vi "Compare to Accel Distances.vi"(5 "dA":dbl, 6 "Sample Period (s)":dbl, 7 "Values":cluster{"accel":dbl, "velocity":dbl}, 8 "Speeds in":T1={"maxV (fps)"=20.0, "Accel Limit (fps^2)"=20.0, "Initial V (fps)"=0.0, "Sample Period (s)"=0.02, "Jerk Limit (fps^3)"=0.0, "Distances"=[]}, 9 "Max Robot Speed":dbl, 10 "Current  Length":dbl, 11 "Total Segment Length":dbl) -> (0 "End Loop":bool, 1 "Ends":cluster{"Accel End":bool, "Decel End":bool}, 2 "Values out":cluster{"accel":dbl, "velocity":dbl}, 3 "Action":enum16{"Const", "Accel", "Decel", "Both"}(ring))   [LabVIEW 2025]
uses:
  Types/Speeds.ctl
panel:
  out "Accel Action":enum16{"Const", "Accel", "Decel", "Both"}(ring)
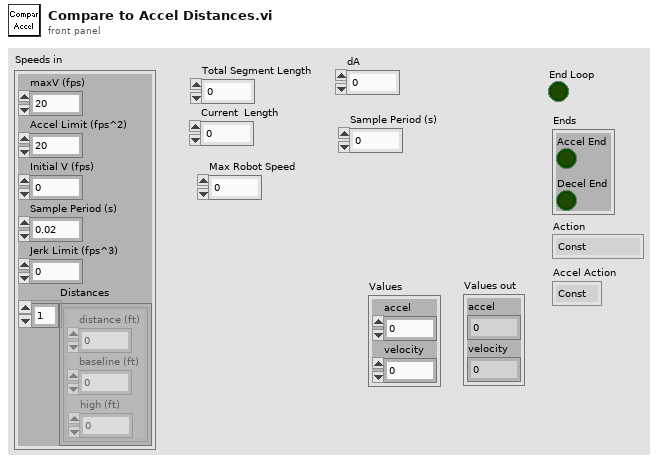
[diagram p1: front panel]
types:
  T1 = typedef "Speeds.ctl" = cluster{"maxV (fps)":dbl, "Accel Limit (fps^2)":dbl, "Initial V (fps)":dbl, "Sample Period (s)":dbl, "Jerk Limit (fps^3)":dbl, "Distances":cluster{"distance (ft)":dbl, "baseline (ft)":dbl, "high (ft)":dbl}[]}
  T2 = cluster{"distance (ft)":dbl, "baseline (ft)":dbl, "high (ft)":dbl}[]
  T3 = cluster{"distance (ft)":dbl, "baseline (ft)":dbl, "high (ft)":dbl}
  T4 = cluster{"distance (ft)":bool, "baseline (ft)":bool, "high (ft)":bool}
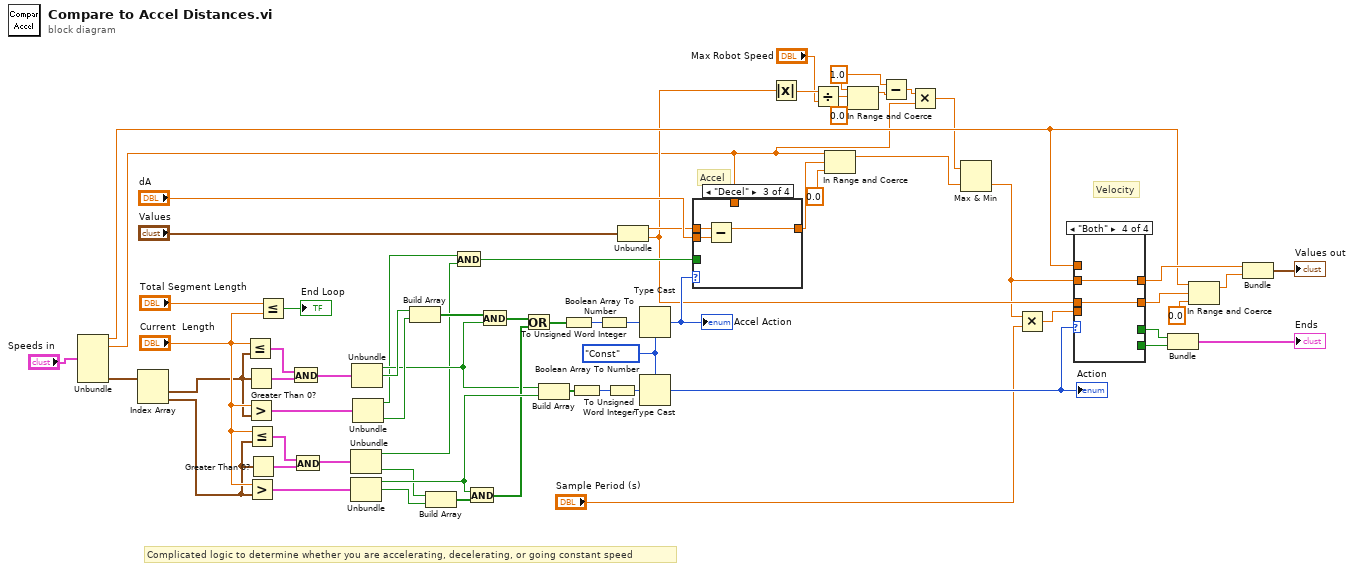
[diagram p0: block diagram]
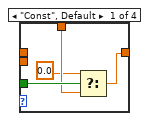
[diagram p2: hidden frame]
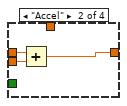
[diagram p3: hidden frame]
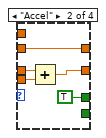
[diagram p6: hidden frame]
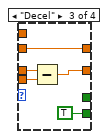
[diagram p7: hidden frame]
diagram:
  w6 = 1.0 ("upper limit")
  w45 = enum16{"Const", "Accel", "Decel", "Both"}."Const" ("Action")
  # "Complicated logic to determine whether you are accelerating, decelerating, or going constant speed"
  # "Accel"
  # "Velocity"
  n1 = Unbundle("Speeds in") -> ("maxV (fps)"=w14:dbl, "Accel Limit (fps^2)"=w4:dbl, "Distances"=w15:T2)  [unwired: 3 out]
  n2 = Index Array(array=w15) -> (element #1=w17:T3, element #2=w16:T3)  [unwired: 2 in]
  n3 = Less Or Equal?(x="Current  Length", y=w17) -> (x <= y?=w62:T4)
  n4 = Greater Than 0?(x=w17) -> (x > 0?=w63:T4)
  n5 = Greater?(x="Current  Length", y=w17) -> (0:w44:T4)
  n6 = Less Or Equal?(x="Current  Length", y=w16) -> (x <= y?=w43:T4)
  n7 = Greater?(x="Current  Length", y=w16) -> (0:w51:T4)
  n8 = Greater Than 0?(x=w16) -> (x > 0?=w42:T4)
  n9 = Less Or Equal?(x="Total Segment Length", y="Current  Length") -> (x <= y?=→"End Loop":bool)
  n10 = And(x=w62, y=w63) -> (x .and. y?=w52:T4)
  n11 = And(x=w43, y=w42) -> (x .and. y?=w39:T4)
  n12 = Unbundle(w39) -> ("distance (ft)"=w19:bool, "high (ft)"=w29:bool)  [unwired: 1 out]
  n13 = Unbundle(w51) -> ("distance (ft)"=w38:bool, "baseline (ft)"=w30:bool)  [unwired: 1 out]
  n14 = Unbundle(w52) -> ("distance (ft)"=w33:bool, "baseline (ft)"=w36:bool)  [unwired: 1 out]
  n15 = Unbundle(w44) -> ("distance (ft)"=w21:bool, "high (ft)"=w40:bool)  [unwired: 1 out]
  n16 = Build Array(w36, w40) -> (w32:bool[])
  n17 = Build Array(w29, w30) -> (w37:bool[])
  n18 = And(x=w21, y=w19) -> (x .and. y?=w20:bool)
  n19 = And(x=w38, y=w37) -> (x .and. y?=w35:bool[])
  n20 = And(x=w32, y=w33) -> (x .and. y?=w31:bool[])
  n21 = Or(x=w31, y=w35) -> (x .or. y?=w34:bool[])
  n22 = Build Array(w33, w38) -> (w53:bool[])
  n23 = Boolean Array To Number(Boolean array=w34) -> (number=w48:u32)
  n24 = Boolean Array To Number(Boolean array=w53) -> (number=w61:u32)
  n25 = To Unsigned Word Integer(number=w48) -> (unsigned 16bit integer=w47:u16)
  n26 = To Unsigned Word Integer(number=w61) -> (unsigned 16bit integer=w50:u16)
  n27 = Unbundle("Values") -> ("accel"=w54:dbl, "velocity"=w12:dbl)
  n28 = Type Cast(type=w45, x=w47) -> (*(type *) &x=w46:enum16{"Const", "Accel", "Decel", "Both"})
  "Accel Action" <- w46
  n29 = Type Cast(type=w45, x=w50) -> (*(type *) &x=w49:enum16{"Const", "Accel", "Decel", "Both"})
  "Action" <- w49
  n30 = case shown="\"Decel\"" w46 {
    tunnel: w54 -> [_ w72 w75 w76]
    tunnel: [w66 w70 w73 w76] -> w24
    tunnel: "dA" -> [_ w71 w74 _]
    tunnel: w4 -> [w68 _ _ _]
    tunnel: w20 -> [w69 _ _ _]
    frame "Const", Default {
      n31 = Select(t=0.0, s=w69, f=w68) -> (s? t:f=w66:dbl)
    }
    frame "Accel" {
      n32 = Add(x=w72, y=w71) -> (x+y=w70:dbl)
    }
    frame "Decel" {
      n33 = Subtract(x=w75, y=w74) -> (x-y=w73:dbl)
    }
    frame "Both" {
    }
  }
  n34 = Absolute Value(x=w12) -> (abs(x)=w11:dbl)
  n35 = Divide(x=w11, y="Max Robot Speed") -> (x/y=w9:dbl)
  n36 = In Range and Coerce(upper limit=w4, x=w24, lower limit=0.0) -> (coerced(x)=w3:dbl)  [unwired: 1 out]
  n37 = In Range and Coerce(upper limit=w6, x=w9, lower limit=0.0) -> (coerced(x)=w7:dbl)  [unwired: 1 out]
  n38 = Subtract(x=w6, y=w7) -> (x-y=w5:dbl)
  n39 = Multiply(x=w5, y=w4) -> (x*y=w2:dbl)
  n40 = Max & Min(x=w2, y=w3) -> (min(x,y)=w1:dbl)  [unwired: 1 out]
  n41 = Multiply(x=w1, y="Sample Period (s)") -> (x*y=w28:dbl)
  n42 = case shown="\"Both\"" w49 {
    tunnel: w12 -> [w77 w83 w88 w90]
    tunnel: [w77 w81 w86 w90] -> w23
    tunnel: w28 -> [_ w82 w87 _]
    tunnel: [_ TRUE _ _] -> w58
    tunnel: [_ _ TRUE _] -> w57
    tunnel: [w78 w79 w84 w89] -> w22
    tunnel: w1 -> [w78 w79 w84 w89]
    tunnel: w14 -> [_ _ _ _]
    frame "Const", Default {
    }
    frame "Accel" {
      n43 = Add(x=w83, y=w82) -> (x+y=w81:dbl)
    }
    frame "Decel" {
      n44 = Subtract(x=w88, y=w87) -> (x-y=w86:dbl)
    }
    frame "Both" {
    }
  }
  n45 = Bundle(w58, w57) -> (→"Ends":cluster{bool, bool})  [unwired: 1 in]
  n46 = In Range and Coerce(upper limit=w14, x=w23, lower limit=0.0) -> (coerced(x)=w13:dbl)  [unwired: 1 out]
  n47 = Bundle(w22, "maxV (fps)"=w13) -> (→"Values out":cluster{dbl, "maxV (fps)":dbl})  [unwired: 1 in]
